vi "_EnumProcesses.vi"(4 "Error In (No Error)":errorcluster, 6 "cb (1024)":u32=1024) -> (0 "Error Out":errorcluster, 1 "lpidProcess":u32[](array[numeric]), 2 "cbNeeded":u32, 3 "#Processes":i32)   [LabVIEW 2018]
uses:
  psapi.dll
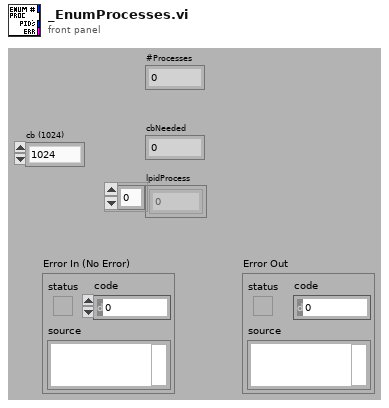
[diagram p1: front panel]
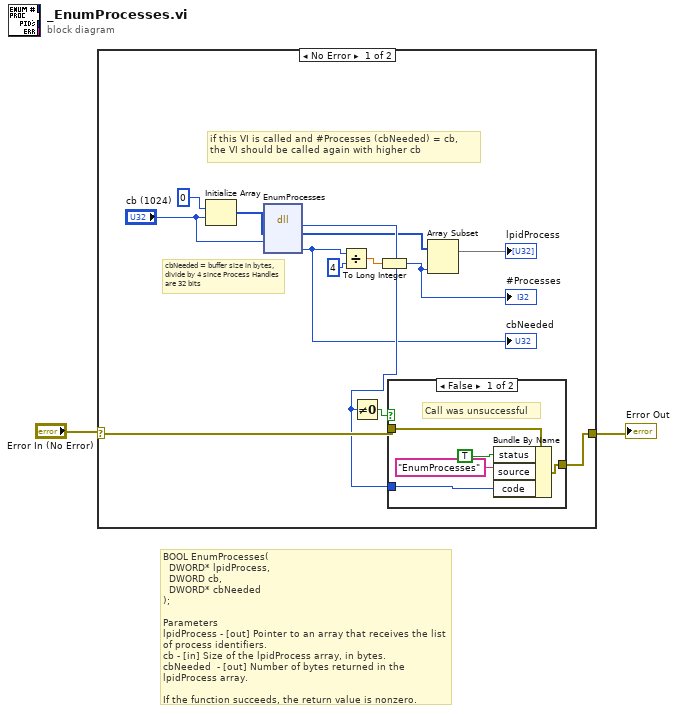
[diagram p0: block diagram]
diagram:
  # "BOOL EnumProcesses(\n  DWORD* lpidProcess,\n  DWORD cb,\n  DWORD* cbNeeded\n);\n\nParameters\nlpidProcess - [out] Pointer to an array that receives the list of process identifiers. \ncb - [in] Size of the lpidProcess array, in bytes. \ncbNeeded  - [out] Number of bytes returned in the lpidProcess array. \n\nIf the function succeeds, the return value is nonzero."
  n1 = case shown="No Error" "Error In (No Error)" {
    selector: "Error In (No Error)" -> [w12 w22]
    tunnel: [w11 w22] -> w1
    frame No Error {
      # "cbNeeded = buffer size in bytes,\ndivide by 4 since Process Handles\nare 32 bits"
      # "if this VI is called and #Processes (cbNeeded) = cb,\nthe VI should be called again with higher cb"
      n2 = Initialize Array(u32 0 ("dimension size"), "cb (1024)") -> (w14:u32[])
      n3 = dll-call lib="psapi.dll" fn="EnumProcesses"("lpidProcess"=w14, "cb"="cb (1024)") -> (w9:i32, "lpidProcess"=w8:u32[], "cbNeeded"=w6:u32)  [unwired: 5 in, 2 out]
      "cbNeeded" <- w6
      n4 = Divide(x=w6, y=4) -> (x/y=w4:dbl)
      n5 = Not Equal To 0?(x=w9) -> (x != 0?=w10:bool)
      n6 = To Long Integer(number=w4) -> (32bit integer=w3:i32)
      "#Processes" <- w3
      n7 = case shown="False" w10 {
        tunnel: w12 -> [w20 w21]
        tunnel: [w17 w21] -> w11
        tunnel: w9 -> [w16 _]
        frame False {
          # "Call was unsuccessful"
          n8 = Bundle By Name(cluster=w20, "status"=TRUE, "source"="EnumProcesses", "code"=w16) -> (w17:errorcluster)
        }
        frame True {
        }
      }
      n9 = Array Subset(array=w8, length=w3) -> (→"lpidProcess":u32[])  [unwired: 1 in]
    }
    frame Error {
    }
  }
  "Error Out" <- w1
